vi "selector_weights.vi"(11 "Selector":T1) -> (3 "Weights":dbl[](array[numeric]))   [LabVIEW 2026]
uses:
  coupling_selector.ctl
panel:
  # "This converts a coupling_selector into a weights vector of 0 or 1 that can be used in distance_processing to select particular row, column or element in the coupling matrix."
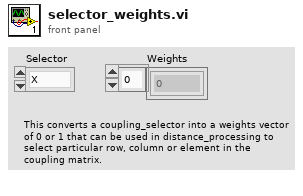
[diagram p1: front panel]
types:
  T1 = typedef "coupling_selector.ctl" = enum16{"X", "Y", "Z", "Vector"}
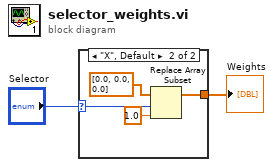
[diagram p0: block diagram]
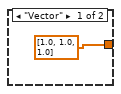
[diagram p2: hidden frame]
diagram:
  n1 = case shown="\"X\", Default" "Selector" {
    selector: "Selector" -> [_ w6]
    tunnel: [dbl[] [1.0, 1.0, 1.0] ("sqrt(x)") w4] -> w2
    frame "Vector" {
    }
    frame "X", Default {
      n2 = Replace Array Subset(array=dbl[] [0.0, 0.0, 0.0] ("sqrt(x)"), new element=1.0 ("new element/subarray"), index=w6) -> (w4:dbl[])
    }
  }
  "Weights" <- w2
